vi "FTW-Reflection-Core-FlatEnum.vi"(7 "Enum Item Name":string, 9 "Enum Type Descriptor":i16[](array[numeric]) format="%04x") -> (6 "Flat Enum Value":string, 8 "Selected Item Index":i32, 10 "Number of Items":i32)   [LabVIEW 2015]
panel:
  # "Inputs"
  # "Outputs"
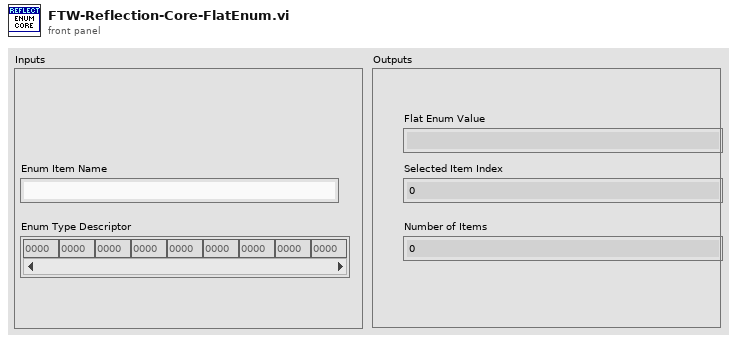
[diagram p1: front panel]
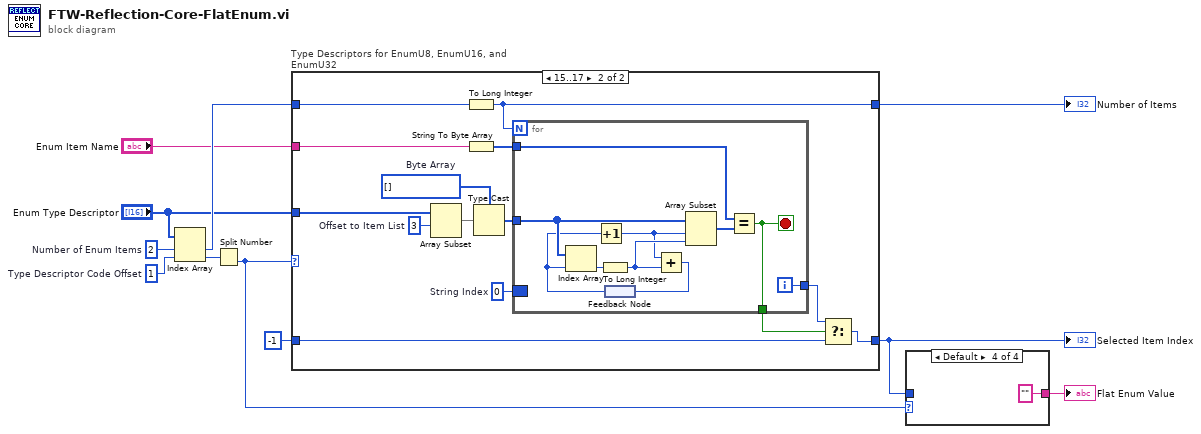
[diagram p0: block diagram]
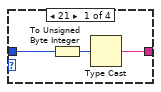
[diagram p2: hidden frame]
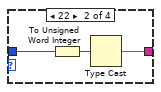
[diagram p3: hidden frame]
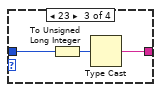
[diagram p4: hidden frame]
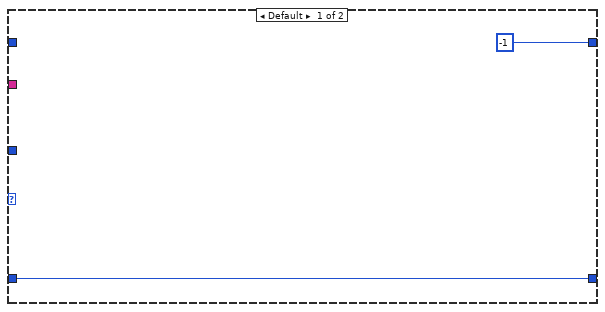
[diagram p5: hidden frame]
diagram:
  w10 = 2  # Number of Enum Items
  w11 = 1  # Type Descriptor Code Offset
  n1 = Index Array(array="Enum Type Descriptor", index #1=w10, index #2=w11) -> (element #1=w9:i16, element #2=w4:i16)
  n2 = Split Number(x=w4) -> (lo(x)=w3:u8)  [unwired: 1 out]
  n3 = case "Type Descriptors for EnumU8, EnumU16, and EnumU32" shown="15..17" w3 {
    tunnel: w9 -> [_ w27]
    tunnel: "Enum Type Descriptor" -> [_ w25]
    tunnel: "Enum Item Name" -> [_ w20]
    tunnel: [w13 w16] -> w2
    tunnel: -1 ("f") -> [w13 w15]
    tunnel: [-1 w14] -> w5
    frame Default {
    }
    frame 21..23 {
      w21 = u8[] []  # Byte Array
      w22 = 0  # String Index
      w23 = 3  # Offset to Item List
      n4 = Array Subset(array=w25, index=w23) -> (w24:i16[])  [unwired: 1 in]
      n5 = To Long Integer(number=w27) -> (32bit integer=w14:i32)
      n6 = String To Byte Array(string=w20) -> (unsigned byte array=w19:u8[])
      n7 = Type Cast(type=w21, x=w24) -> (*(type *) &x=w26:u8[])
      n8 = for {
        N: w14 -> [_]
        tunnel: w26 -> [w35]
        border: w22 -> [_]
        tunnel: w19 -> [w29]
        tunnel: [w32] -> w17
        tunnel: [w28] -> w18
        i -> [w32]
        stop <- w28 stop-if-true
        n9 = feedback #1() -> (w34:i32)
        n10 = Index Array(array=w35, index=w34) -> (element=w37:u8)
        n11 = Increment(x=w34) -> (x+1=w30:i32)
        n12 = To Long Integer(number=w37) -> (32bit integer=w33:i32)
        n13 = Add(x=w30, y=w33) -> (x+y=w36:i32)
        n14 = feedback-in #1(w36) -> ()
        n15 = Array Subset(array=w35, index=w30, length=w33) -> (w31:u8[])
        n16 = Equal?(x=w29, y=w31) -> (x = y?=w28:bool)
      }
      n17 = Select(t=w17, s=w18, f=w15) -> (s? t:f=w16:i32)
    }
  }
  "Selected Item Index" <- w2
  "Number of Items" <- w5
  n18 = case shown="Default" w3 {
    tunnel: w2 -> [w38 w41 w44 _]
    tunnel: [w39 w42 w45 ""] -> w1
    frame 21 {
      n19 = To Unsigned Byte Integer(number=w38) -> (unsigned 8bit integer=w40:u8)
      n20 = Type Cast(x=w40) -> (*(type *) &x=w39:string)  [unwired: 1 in]
    }
    frame 22 {
      n21 = To Unsigned Word Integer(number=w41) -> (unsigned 16bit integer=w43:u16)
      n22 = Type Cast(x=w43) -> (*(type *) &x=w42:string)  [unwired: 1 in]
    }
    frame 23 {
      n23 = To Unsigned Long Integer(number=w44) -> (unsigned 32bit integer=w46:u32)
      n24 = Type Cast(x=w46) -> (*(type *) &x=w45:string)  [unwired: 1 in]
    }
    frame Default {
    }
  }
  "Flat Enum Value" <- w1
